vi "Write Search.vi"(10 "Search":refnum<class "Search.lvclass">, 11 "Node in":refnum<class "Node.lvclass">) -> (3 "Node out":refnum<class "Node.lvclass">)   [LabVIEW 2016, in "Node.lvclass"]
uses:
  Node.lvclass
  Search/Search.lvclass
  Node.lvclass/Node.ctl
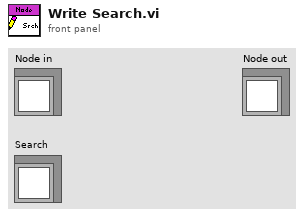
[diagram p1: front panel]
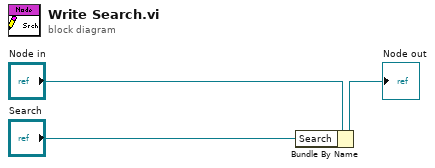
[diagram p0: block diagram]
diagram:
  n1 = Bundle By Name(cluster="Node in", "Search"="Search") -> (→"Node out":refnum<class "Node.lvclass">)
